vi "LINC Get Item Format.vi"(8 "error in (no error)":errorcluster, 10 "control reference":refnum<vi>, 11 "LINC session":refnum<class "LINC.lvclass">) -> (0 "error out":errorcluster, 1 "item name":string, 2 "item format":T1)   [LabVIEW 2018, in "STEPkgDriver_LINC.lvlib" / "LINC.lvclass"]
uses:
  LINC.lvclass
  STEPkgDriver_LINC.lvlib
  LINC Format Prototype.ctl
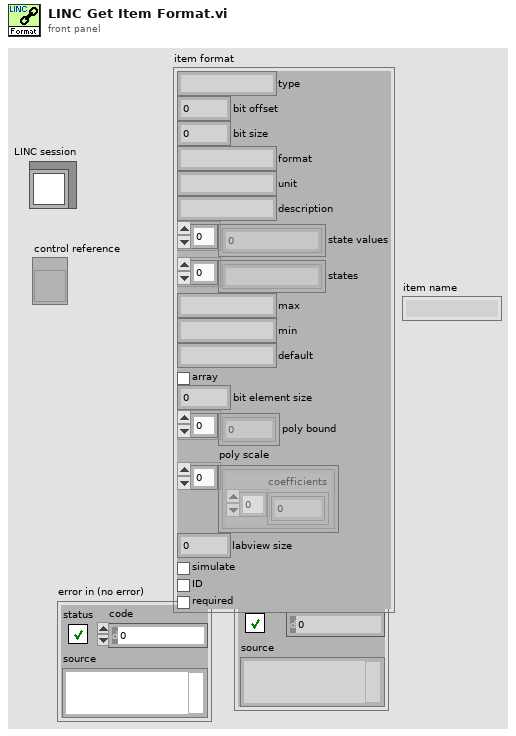
[diagram p1: front panel]
types:
  T1 = typedef "STEPkgDriver_LINC.lvlib/LINC Format Prototype.ctl" = cluster{"type":string, "bit offset":i32, "bit size":i32, "format":string, "unit":string, "description":string, "state values":i64[], "states":string[], "max":string, "min":string, "default":string, "array":bool, "bit element size":i32, "poly bound":dbl[], "poly scale":cluster{"coefficients":dbl[]}[], "labview size":i32, "simulate":bool, "ID":bool, "required":bool}
  T2 = cluster{"type":string, "bits":i32, "elements":i32, "unit":string, "poly scale":dbl[], "ID":bool, "REQUIRED":bool}
  T3 = cluster{"type":string, "bits":i32, "value":string, "array":bool}
  T4 = typedef "LVStringsAndValuesArrayTypeDef.ctl" = cluster{"String":string, "Value":ext}[]
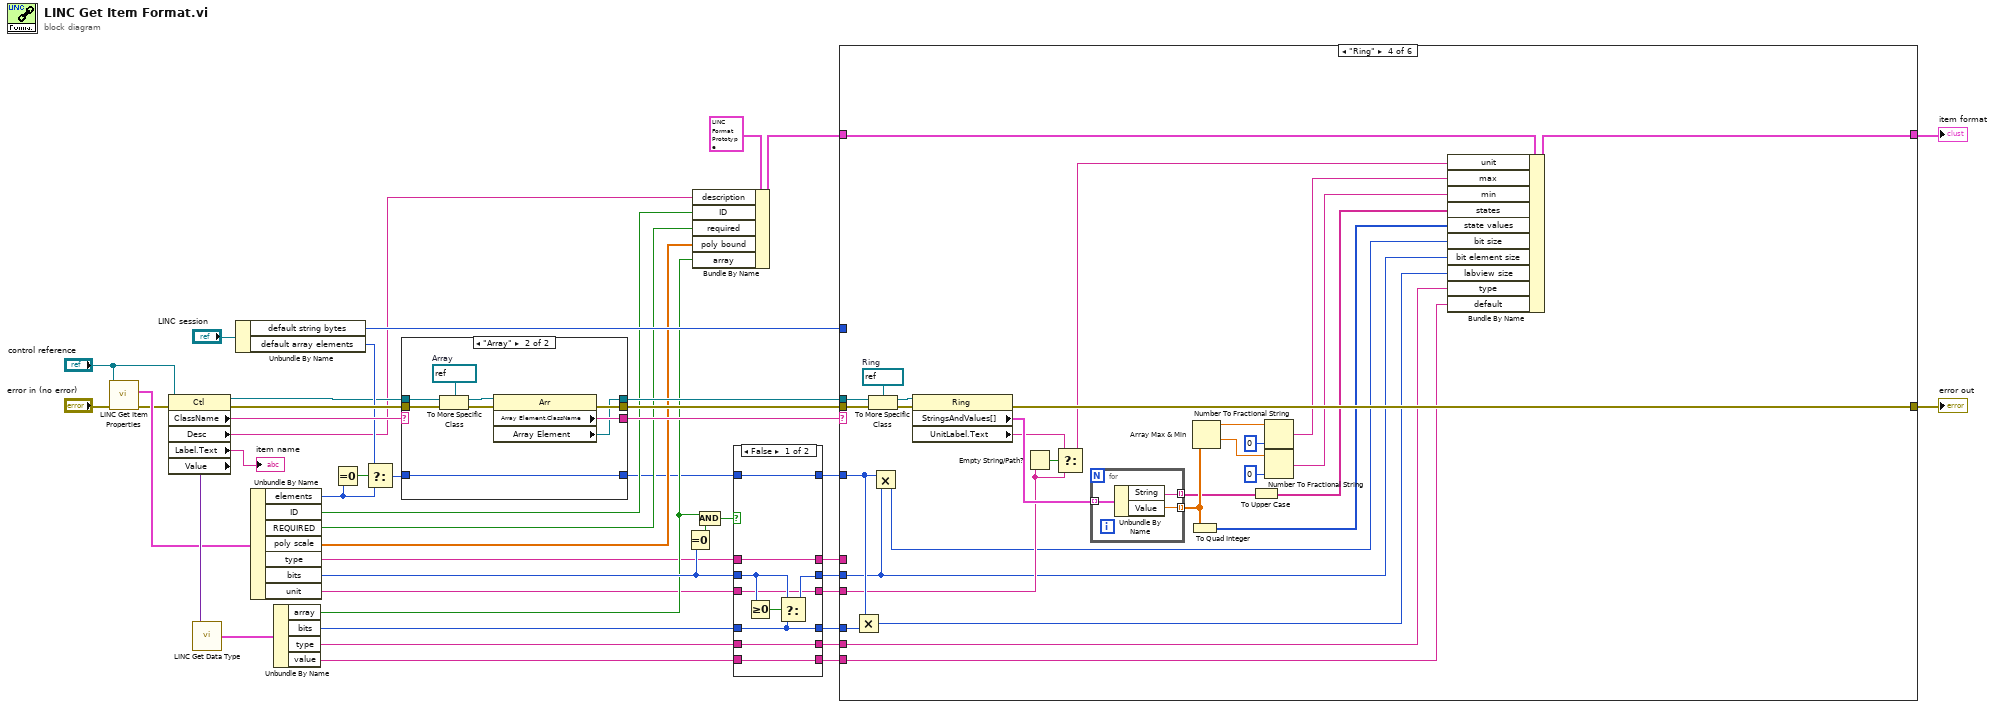
[diagram p0: block diagram]
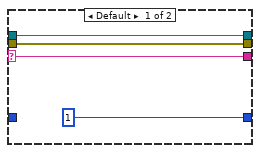
[diagram p3: hidden frame]
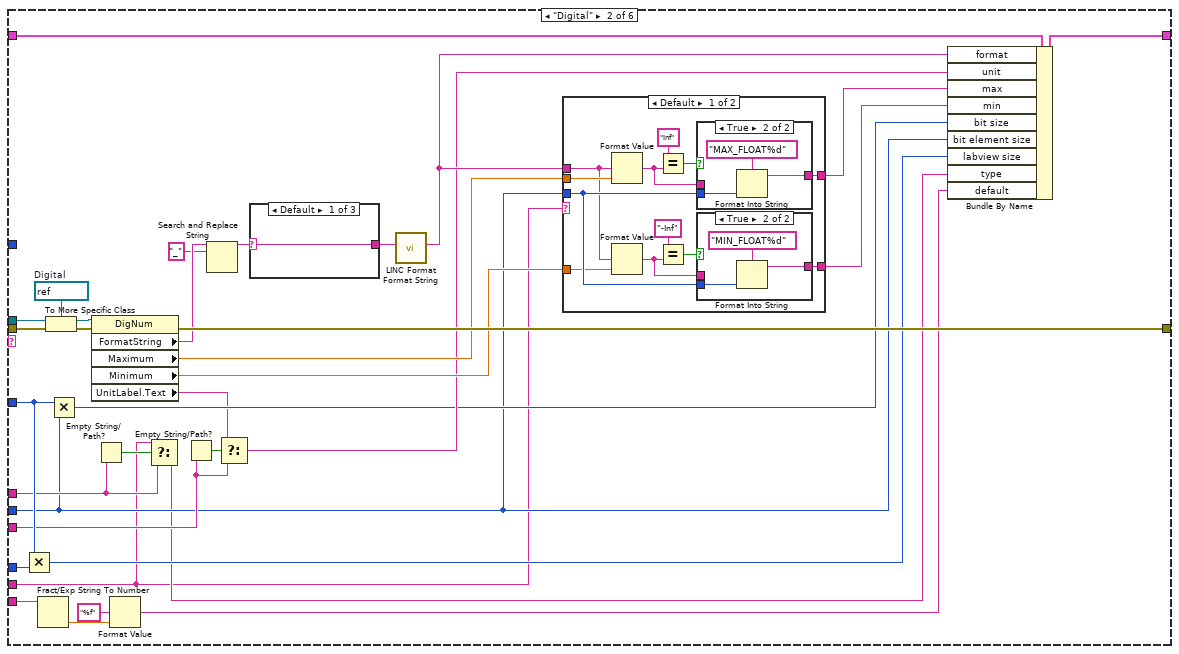
[diagram p5: hidden frame]
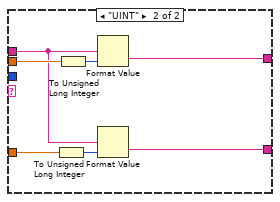
[diagram p8: hidden frame]
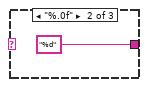
[diagram p9: hidden frame]
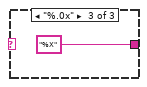
[diagram p10: hidden frame]
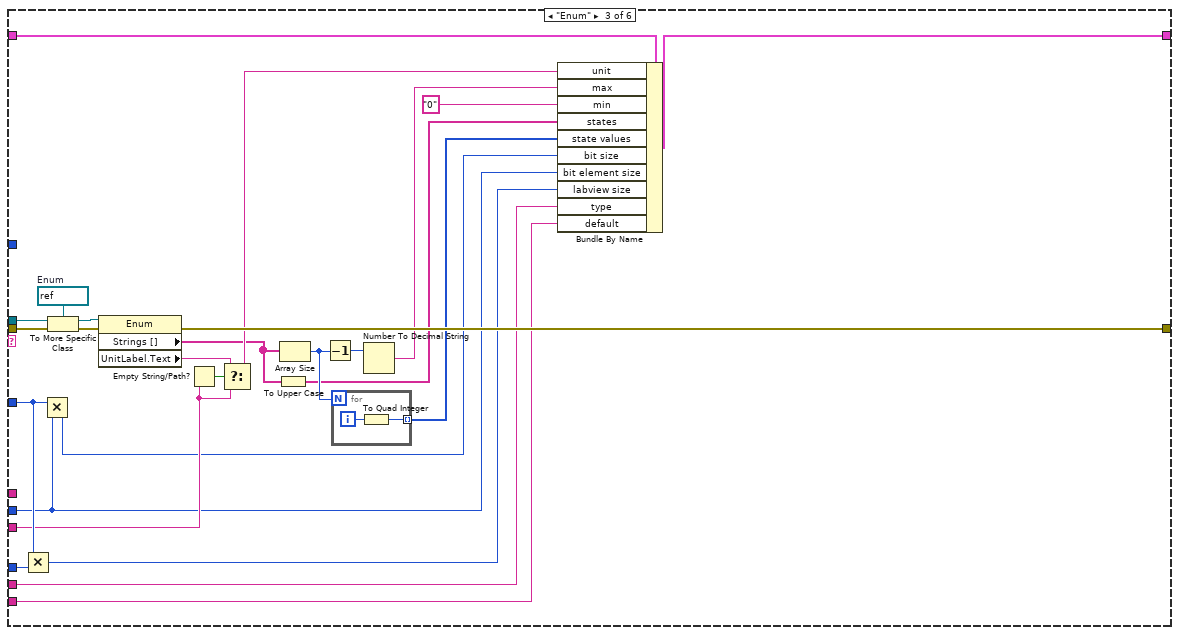
[diagram p11: hidden frame]
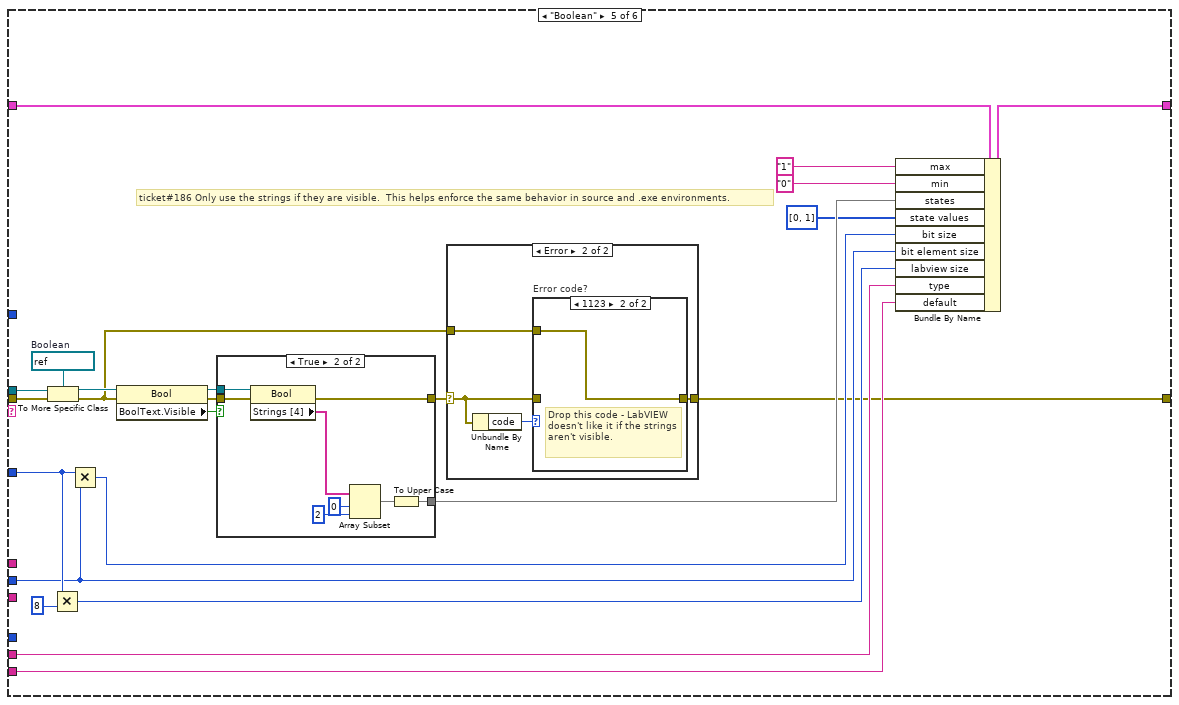
[diagram p12: hidden frame]
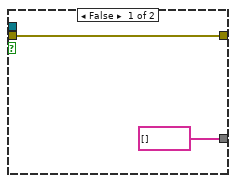
[diagram p15: hidden frame]
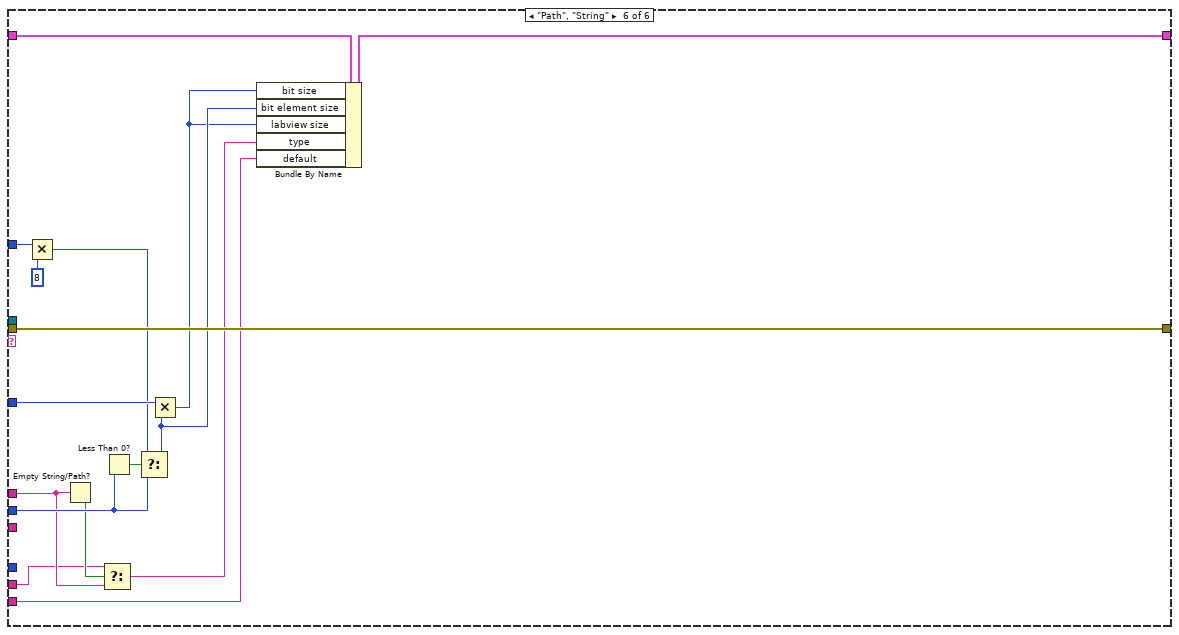
[diagram p16: hidden frame]
diagram:
  n1 = call "LINC Get Item Properties.vi"("error in (no error)"="error in (no error)", "control reference"="control reference") -> ("error out"=w19:errorcluster, "properties"=w23:T2)  [unwired: 8 in]
  n2 = property class="Ctl"(reference="control reference", error in=w19) -> (reference out=w31:refnum<vi>, error out=w37:errorcluster, "ClassName"=w44:string, "Desc"=w28:string, "Label.Text"=→"item name":string, "Value"=w26:variant)
  n3 = call "LINC Get Data Type.vi"("variant"=w26) -> ("properties"=w25:T3)
  n4 = Unbundle By Name("LINC session") -> ("default string bytes"=w33:i32, "default array elements"=w32:i32)
  n5 = Unbundle By Name(w23) -> ("elements"=w22:i32, "ID"=w20:bool, "REQUIRED"=w16:bool, "poly scale"=w21:dbl[], "type"=w9:string, "bits"=w15:i32, "unit"=w7:string)
  n6 = Unbundle By Name(w25) -> ("array"=w14:bool, "bits"=w24:i32, "type"=w5:string, "value"=w3:string)
  n7 = Equal To 0?(x=w22) -> (x = 0?=w40:bool)
  n8 = Select(t=w32, s=w40, f=w22) -> (s? t:f=w39:i32)
  n9 = case shown="\"Array\"" w44 {
    selector: w44 -> [w48 _]
    tunnel: [w48 w52] -> w43
    tunnel: w37 -> [w47 w54]
    tunnel: [w47 w51] -> w36
    tunnel: w31 -> [w46 w53]
    tunnel: [w46 w50] -> w42
    tunnel: w39 -> [_ w49]
    tunnel: [1 ("default array elements") w49] -> w11
    frame Default {
    }
    frame "Array" {
      w57 = refnum<vi> refnum  # Array
      n10 = To More Specific Class(target class=w57, reference=w53, error in=w54) -> (specific class reference=w55:refnum<vi>, error out=w56:errorcluster)
      n11 = property class="Arr"(reference=w55, error in=w56) -> (error out=w51:errorcluster, "Array Element.ClassName"=w52:string, "Array Element"=w50:refnum<vi>)  [unwired: 1 out]
    }
  }
  n12 = Equal To 0?(x=w15) -> (x = 0?=w13:bool)
  n13 = Bundle By Name(cluster=T1 {"type"="", "bit offset"=0, "bit size"=0, "format"="", "unit"="", "description"="", "state values"=[], "states"=[], "max"="", "min"="", "default"="", "array"=FALSE, "bit element size"=0, "poly bound"=[], "poly scale"=[], "labview size"=0, "simulate"=FALSE, "ID"=FALSE, "required"=FALSE} ("data"), "description"=w28, "ID"=w20, "required"=w16, "poly bound"=w21, "array"=w14) -> (w29:T1)
  n14 = And(x=w14, y=w13) -> (x .and. y?=w12:bool)
  n15 = case shown="False" w12 {
    tunnel: [w65 w67] -> w41
    tunnel: w24 -> [w58 w67]
    tunnel: w15 -> [w64 _]
    tunnel: w11 -> [w63 _]
    tunnel: [w63 _] -> w10
    tunnel: w9 -> [w62 w71]
    tunnel: [w62 w71] -> w8
    tunnel: w7 -> [w61 w70]
    tunnel: [w61 w70] -> w6
    tunnel: w5 -> [w60 w69]
    tunnel: [w60 w69] -> w4
    tunnel: w3 -> [w59 w68]
    tunnel: [w59 w68] -> w2
    tunnel: [w58 _] -> w1
    frame False {
      n16 = Greater Or Equal To 0?(x=w64) -> (x >= 0?=w66:bool)
      n17 = Select(t=w64, s=w66, f=w58) -> (s? t:f=w65:i32)
    }
    frame True {
    }
  }
  n18 = case shown="\"Ring\"" w43 {
    tunnel: w42 -> [_ w105 w161 w193 w220 _]
    tunnel: w36 -> [w73 w103 w159 w190 w219 w254]
    tunnel: w33 -> [_ _ _ _ _ w253]
    tunnel: [w73 w102 w158 w189 w199 w254] -> w35
    tunnel: w41 -> [_ w79 w141 w171 w209 w248]
    tunnel: w10 -> [_ w98 w155 w183 w218 w251]
    tunnel: w1 -> [_ w99 w154 w182 _ _]
    tunnel: w8 -> [_ w94 _ _ _ w246]
    tunnel: w4 -> [_ w74 w139 w169 w207 w245]
    tunnel: w2 -> [_ w92 w138 w168 w206 w239]
    tunnel: w29 -> [w72 w88 w153 w181 w216 w244]
    tunnel: [w72 w87 w152 w180 w215 w243] -> w27
    tunnel: w6 -> [_ w84 w149 w177 _ _]
    frame Default {
    }
    frame "Digital" {
      w107 = refnum<vi> refnum  # Digital
      n19 = Multiply(x=w98, y=w99) -> (x*y=w78:i32)
      n20 = Fract/Exp String To Number(string=w92) -> (number=w93:dbl)  [unwired: 3 in, 1 out]
      n21 = To More Specific Class(target class=w107, reference=w105, error in=w103) -> (specific class reference=w104:refnum<vi>, error out=w106:errorcluster)
      n22 = Multiply(x=w98, y=w79) -> (x*y=w80:i32)
      n23 = property class="DigNum"(reference=w104, error in=w106) -> (error out=w102:errorcluster, "FormatString"=w101:string, "Maximum"=w97:dbl, "Minimum"=w96:dbl, "UnitLabel.Text"=w75:string)  [unwired: 1 out]
      n24 = Empty String/Path?(string/path=w94) -> (empty?=w95:bool)
      n25 = Format Value(format string="%f", value (0)=w93) -> (output string=w76:string)  [unwired: 1 out]
      n26 = Select(t=w74, s=w95, f=w94) -> (s? t:f=w77:string)
      n27 = Empty String/Path?(string/path=w84) -> (empty?=w86:bool)
      n28 = Search and Replace String(input string=w101, search string="_") -> (result string=w90:string)  [unwired: 1 in, 8 out]
      n29 = Select(t=w75, s=w86, f=w84) -> (s? t:f=w83:string)
      n30 = case shown="Default" w90 {
        selector: w90 -> [w135 _ _]
        tunnel: [w135 "%d" ("t") "%X" ("t")] -> w89
        frame Default {
        }
        frame "%.0f" {
        }
        frame "%.0x" {
        }
      }
      n31 = call "LINC Format Format String.vi"("format in"=w89) -> ("format out"=w85:string)  [unwired: 10 in]
      n32 = case shown="Default" w74 {
        tunnel: [w116 w131] -> w82
        tunnel: [w112 w130] -> w81
        tunnel: w79 -> [w111 _]
        tunnel: w97 -> [w110 w134]
        tunnel: w96 -> [w109 w133]
        tunnel: w85 -> [w108 w132]
        frame Default {
          n33 = Format Value(format string=w108, value (0)=w110) -> (output string=w117:string)  [unwired: 1 out]
          n34 = Format Value(format string=w108, value (0)=w109) -> (output string=w115:string)  [unwired: 1 out]
          n35 = Equal?(x="Inf", y=w117) -> (x = y?=w118:bool)
          n36 = Equal?(x="-Inf", y=w115) -> (x = y?=w114:bool)
          n37 = case shown="True" w118 {
            tunnel: w111 -> [_ w126]
            tunnel: w117 -> [w124 _]
            tunnel: [w124 w125] -> w116
            frame False {
            }
            frame True {
              n38 = Format Into String(format string="MAX_FLOAT%d", w126) -> (resulting string=w125:string)  [unwired: 2 in, 1 out]
            }
          }
          n39 = case shown="True" w114 {
            tunnel: w111 -> [_ w122]
            tunnel: w115 -> [w120 _]
            tunnel: [w120 w121] -> w112
            frame False {
            }
            frame True {
              n40 = Format Into String(format string="MIN_FLOAT%d", w122) -> (resulting string=w121:string)  [unwired: 2 in, 1 out]
            }
          }
        }
        frame "UINT" {
          n41 = To Unsigned Long Integer(number=w133) -> (unsigned 32bit integer=w128:u32)
          n42 = To Unsigned Long Integer(number=w134) -> (unsigned 32bit integer=w129:u32)
          n43 = Format Value(format string=w132, value (0)=w129) -> (output string=w131:string)  [unwired: 1 out]
          n44 = Format Value(format string=w132, value (0)=w128) -> (output string=w130:string)  [unwired: 1 out]
        }
      }
      n45 = Bundle By Name(cluster=w88, "format"=w85, "unit"=w83, "max"=w82, "min"=w81, "bit size"=w80, "bit element size"=w79, "labview size"=w78, "type"=w77, "default"=w76) -> (w87:T1)
    }
    frame "Enum" {
      w163 = refnum<vi> refnum  # Enum
      n46 = Multiply(x=w155, y=w154) -> (x*y=w140:i32)
      n47 = Multiply(x=w155, y=w141) -> (x*y=w142:i32)
      n48 = To More Specific Class(target class=w163, reference=w161, error in=w159) -> (specific class reference=w160:refnum<vi>, error out=w162:errorcluster)
      n49 = property class="Enum"(reference=w160, error in=w162) -> (error out=w158:errorcluster, "Strings []"=w146:string[], "UnitLabel.Text"=w150:string)  [unwired: 1 out]
      n50 = Empty String/Path?(string/path=w149) -> (empty?=w151:bool)
      n51 = Select(t=w150, s=w151, f=w149) -> (s? t:f=w148:string)
      n52 = To Upper Case(1:w146) -> (0:w145:string[])
      n53 = Array Size(array=w146) -> (size(s)=w156:i32)
      n54 = Decrement(x=w156) -> (x-1=w157:i32)
      n55 = for {
        N: w156 -> [_]
        tunnel: [w164] -> w144 mode=indexing
        i -> [w165]
        n56 = To Quad Integer(1:w165) -> (0:w164:i64)
      }
      n57 = Number To Decimal String(number=w157) -> (decimal integer string=w147:string)  [unwired: 1 out]
      n58 = Bundle By Name(cluster=w153, "unit"=w148, "max"=w147, "min"="0" ("output string"), "states"=w145, "state values"=w144, "bit size"=w142, "bit element size"=w141, "labview size"=w140, "type"=w139, "default"=w138) -> (w152:T1)
    }
    frame "Ring" {
      w195 = refnum<vi> refnum  # Ring
      n59 = Multiply(x=w183, y=w182) -> (x*y=w170:i32)
      n60 = To More Specific Class(target class=w195, reference=w193, error in=w190) -> (specific class reference=w192:refnum<vi>, error out=w194:errorcluster)
      n61 = Multiply(x=w183, y=w171) -> (x*y=w172:i32)
      n62 = property class="Ring"(reference=w192, error in=w194) -> (error out=w189:errorcluster, "StringsAndValues[]"=w191:T4, "UnitLabel.Text"=w178:string)  [unwired: 1 out]
      n63 = Empty String/Path?(string/path=w177) -> (empty?=w179:bool)
      n64 = Select(t=w178, s=w179, f=w177) -> (s? t:f=w176:string)
      n65 = for {
        tunnel: w191 -> [w198] mode=indexing
        tunnel: [w197] -> w167 mode=indexing
        tunnel: [w196] -> w184 mode=indexing
        n66 = Unbundle By Name(w198) -> ("String"=w197:string, "Value"=w196:ext)
      }
      n67 = To Quad Integer(1:w184) -> (0:w173:i64[])
      n68 = Array Max & Min(array=w184) -> (max value=w188:ext, min value=w185:ext)  [unwired: 2 out]
      n69 = To Upper Case(1:w167) -> (0:w166:string[])
      n70 = Number To Fractional String(number=w188, precision (6)=i16 0) -> (F-format string=w175:string)  [unwired: 2 out]
      n71 = Number To Fractional String(number=w185, precision (6)=i16 0) -> (F-format string=w174:string)  [unwired: 2 out]
      n72 = Bundle By Name(cluster=w181, "unit"=w176, "max"=w175, "min"=w174, "states"=w166, "state values"=w173, "bit size"=w172, "bit element size"=w171, "labview size"=w170, "type"=w169, "default"=w168) -> (w180:T1)
    }
    frame "Boolean" {
      w221 = refnum<vi> refnum  # Boolean
      # "ticket#186 Only use the strings if they are visible.  This helps enforce the same behavior in source and .exe environments."
      n73 = To More Specific Class(target class=w221, reference=w220, error in=w219) -> (specific class reference=w205:refnum<vi>, error out=w200:errorcluster)
      n74 = Multiply(x=w218, y=8 ("bits")) -> (x*y=w208:i32)
      n75 = Multiply(x=w218, y=w209) -> (x*y=w210:i32)
      n76 = property class="Bool"(reference=w205, error in=w200) -> (reference out=w203:refnum<vi>, error out=w204:errorcluster, "BoolText.Visible"=w202:bool)
      n77 = case shown="True" w202 {
        tunnel: [string[] [] w234] -> w212
        tunnel: w204 -> [w230 w233]
        tunnel: [w230 w231] -> w201
        tunnel: w203 -> [_ w232]
        frame False {
        }
        frame True {
          n78 = property class="Bool"(reference=w232, error in=w233) -> (error out=w231:errorcluster, "Strings [4]"=w238:string[])  [unwired: 1 out]
          n79 = Array Subset(array=w238, index=0, length=2) -> (w235:string[])
          n80 = To Upper Case(1:w235) -> (0:w234:string[])
        }
      }
      n81 = case shown="Error" w201 {
        selector: w201 -> [w222 w223]
        tunnel: [w222 w225] -> w199
        tunnel: w200 -> [_ w224]
        frame No Error {
        }
        frame Error {
          n82 = Unbundle By Name(w223) -> ("code"=w226:i32)
          n83 = case "Error code?" shown="1123" w226 {
            tunnel: [w227 w228] -> w225
            tunnel: w224 -> [_ w228]
            tunnel: w223 -> [w227 _]
            frame Default {
            }
            frame 1123 {
              # "Drop this code - LabVIEW doesn't like it if the strings aren't visible."
            }
          }
        }
      }
      n84 = Bundle By Name(cluster=w216, "max"="1" ("output string"), "min"="0" ("output string"), "states"=w212, "state values"=u32[] [0, 1], "bit size"=w210, "bit element size"=w209, "labview size"=w208, "type"=w207, "default"=w206) -> (w215:T1)
    }
    frame "Path", "String" {
      n85 = Multiply(x=w253, y=8) -> (x*y=w249:i32)
      n86 = Empty String/Path?(string/path=w246) -> (empty?=w247:bool)
      n87 = Select(t=w245, s=w247, f=w246) -> (s? t:f=w240:string)
      n88 = Less Than 0?(x=w248) -> (x < 0?=w250:bool)
      n89 = Select(t=w249, s=w250, f=w248) -> (s? t:f=w242:i32)
      n90 = Multiply(x=w251, y=w242) -> (x*y=w241:i32)
      n91 = Bundle By Name(cluster=w244, "bit size"=w241, "bit element size"=w242, "labview size"=w241, "type"=w240, "default"=w239) -> (w243:T1)
    }
  }
  "error out" <- w35
  "item format" <- w27
